vi "12-sub.vi"(11 "Number":i32=5) -> (0 "number of divisors":i32, 3 "Divisors":set{i32}(c389))   [LabVIEW 2021]
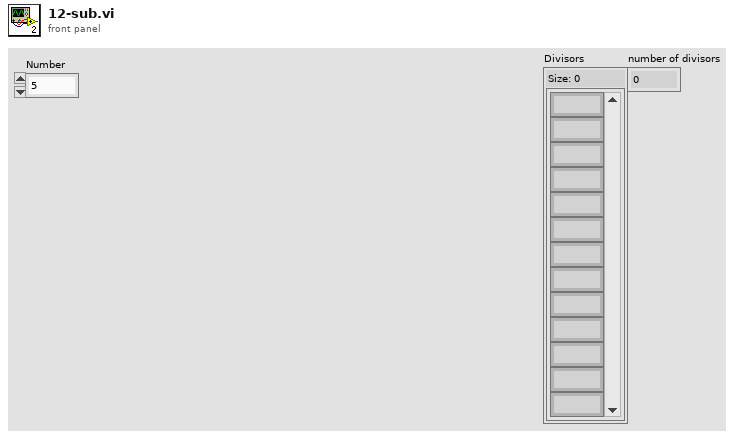
[diagram p1: front panel]
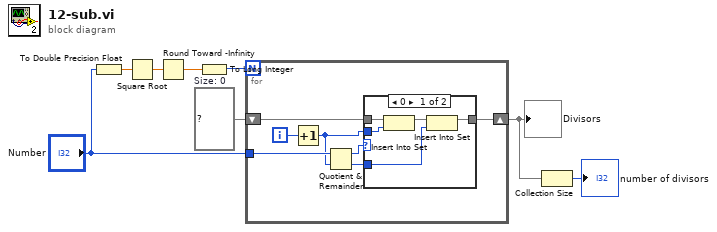
[diagram p0: block diagram]
diagram:
  w6 = set{i32} {}  # Size: 0
  n1 = To Double Precision Float(number="Number") -> (double precision float=w3:dbl)
  n2 = Square Root(x=w3) -> (sqrt(x)=w8:dbl)
  n3 = Round Toward -Infinity(1:w8) -> (0:w5:dbl)
  n4 = To Long Integer(number=w5) -> (32bit integer=w4:i32)
  n5 = for {
    N: w4 -> [_]
    tunnel: "Number" -> [w15]
    shift-right: [w11] -> w2
    shift-left: w6 -> [w10]
    i -> [w13]
    n6 = Increment(x=w13) -> (x+1=w9:i32)
    n7 = Quotient & Remainder(x=w15, y=w9) -> (x-y*floor(x/y)=w14:i32, floor(x/y)=w12:i32)
    n8 = case shown="0" w14 {
      tunnel: w9 -> [w19 _]
      tunnel: w12 -> [w18 _]
      tunnel: [w17 w21] -> w11
      tunnel: w10 -> [w16 w21]
      frame 0 {
        n9 = Insert Into Set(10:w19, 11:w16) -> (3:w20:set{i32})  [unwired: 1 out]
        n10 = Insert Into Set(10:w18, 11:w20) -> (3:w17:set{i32})  [unwired: 1 out]
      }
      frame Default {
      }
    }
  }
  "Divisors" <- w2
  n11 = Collection Size(1:w2) -> (0:→"number of divisors":i32)
